vi "Handshake.vi"(6 "TCP Connection":refnum<k5>, 8 "error in (no error)":errorcluster, 11 "Websocket Client in":refnum<class "Websocket Client.lvclass">) -> (0 "error out":errorcluster, 3 "Websocket Client out":refnum<class "Websocket Client.lvclass">)   [LabVIEW 2020, in "Stream-Websocket.lvlib" / "Websocket Client.lvclass"]
uses:
  Websocket Client.lvclass
  Websocket Client.lvclass/Websocket Client.ctl
  <vilib>/IlluminatedG/IG HTTP Utils/HTTP Utils/Request/Request.lvclass
  Stream-Websocket.lvlib
  <vilib>/IlluminatedG/IG HTTP Utils/HTTP Utils/Response/Response.lvclass
  WebSocketUpgradeResponse/WebSocketUpgradeResponse.lvclass
  C:/Program Files (x86)/National Instruments/LabVIEW 2020/vi.lib/IlluminatedG/IG HTTP Utils/HTTP Utils/Response/Response.lvclass
  C:/dev/IlluminatedG/lv-stream-websocket/Stream-Websocket/WebSocketUpgradeResponse/WebSocketUpgradeResponse.lvclass
panel:
  out "WebSocket Response":refnum<class "WebSocketUpgradeResponse.lvclass">
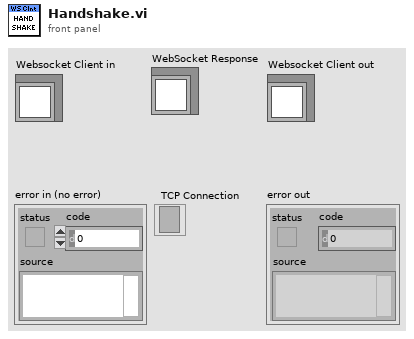
[diagram p1: front panel]
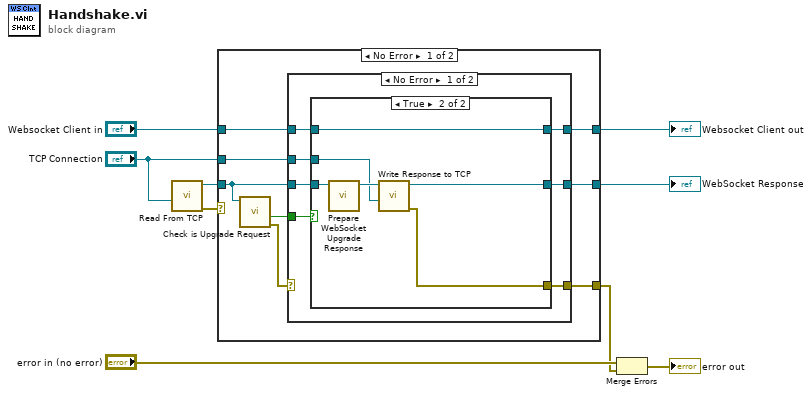
[diagram p0: block diagram]
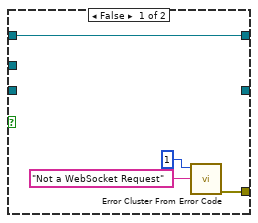
[diagram p2: hidden frame]
diagram:
  n1 = call <vilib>:"Read From TCP.vi"("TCP Connection"="TCP Connection") -> ("error out"=w9:errorcluster, "Request out"=w8:refnum<class "Request.lvclass">)  [unwired: 9 in]
  n2 = case shown="No Error" w9 {
    selector: w9 -> [_ w38]
    tunnel: w8 -> [w16 _]
    tunnel: [w14 w38] -> w5
    tunnel: [w13 _] -> w7
    tunnel: "Websocket Client in" -> [w12 w37]
    tunnel: [w11 w37] -> w2
    tunnel: "TCP Connection" -> [w10 _]
    frame No Error {
      n3 = call "Check is Upgrade Request.vi"("Request in"=w16) -> ("error out"=w15:errorcluster, "Upgrade Request?"=w17:bool)  [unwired: 7 in, 2 out]
      n4 = case shown="No Error" w15 {
        selector: w15 -> [_ w36]
        tunnel: w16 -> [w23 _]
        tunnel: w17 -> [w24 _]
        tunnel: [w22 w36] -> w14
        tunnel: [w21 _] -> w13
        tunnel: w12 -> [w20 w35]
        tunnel: [w19 w35] -> w11
        tunnel: w10 -> [w18 _]
        frame No Error {
          n5 = case shown="True" w24 {
            tunnel: w23 -> [_ w34]
            tunnel: [w26 w29] -> w22
            tunnel: [_ w30] -> w21
            tunnel: w20 -> [w25 w33]
            tunnel: [w25 w33] -> w19
            tunnel: w18 -> [_ w31]
            frame False {
              n6 = call <vilib>:"Error Cluster From Error Code.vi"("error message (\"\")"="Not a WebSocket Request" ("error message (\"\")"), "error code (0)"=1) -> ("error out"=w26:errorcluster)  [unwired: 7 in]
            }
            frame True {
              n7 = call "Prepare WebSocket Upgrade Response.vi"("Request"=w34) -> ("WebSocket Response"=w32:refnum<class "WebSocketUpgradeResponse.lvclass">)  [unwired: 10 in]
              n8 = call <vilib>:"Write Response to TCP.vi"("TCP Connection"=w31, "Response in"=w32) -> ("error out"=w29:errorcluster, "Response out"=w30:refnum<class "WebSocketUpgradeResponse.lvclass">)  [unwired: 8 in]
            }
          }
        }
        frame Error {
        }
      }
    }
    frame Error {
    }
  }
  "Websocket Client out" <- w2
  "WebSocket Response" <- w7
  n9 = Merge Errors("error in (no error)", w5) -> (→"error out":errorcluster)
